vi "IMU_Single_Read_Data.vi"(8 "error in (no error)":errorcluster caption="Fehler (Eingang, kein Fehler)", 9 "Delay (ms)":u32, 11 "VISA resource name IN":refnum<visa-resource-name>) -> (0 "error out":errorcluster caption="Fehler (Ausgang)", 2 "Received Raw Data Byte-Array U8":u8[](array[numeric]), 3 "VISA resource name OUT":refnum<visa-resource-name>)   [LabVIEW 2017]
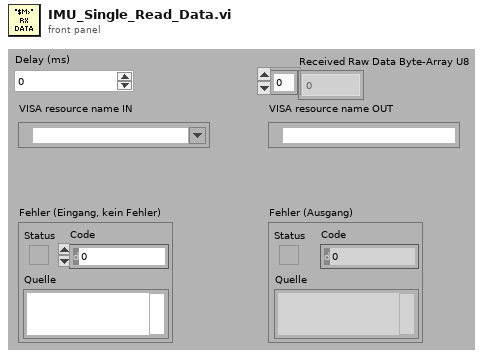
[diagram p1: front panel]
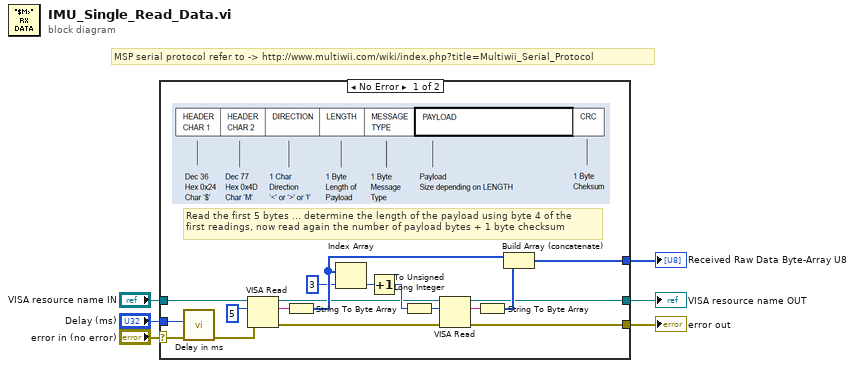
[diagram p0: block diagram]
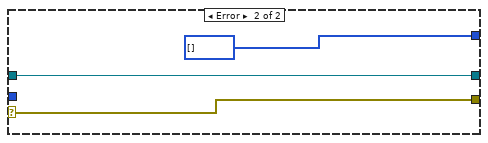
[diagram p2: hidden frame]
diagram:
  # "MSP serial protocol refer to -> http://www.multiwii.com/wiki/index.php?title=Multiwii_Serial_Protocol"
  n1 = case shown="No Error" "error in (no error)" {
    selector: "error in (no error)" -> [w24 w26]
    tunnel: "VISA resource name IN" -> [w9 w27]
    tunnel: [w11 w26] -> w5
    tunnel: [w10 w27] -> w4
    tunnel: [w8 u8[] [] ("Received Raw Data Byte-Array U8 2")] -> w3
    tunnel: "Delay (ms)" -> [w23 _]
    frame No Error {
      # "Read the first 5 bytes ... determine the length of the payload using byte 4 of the\nfirst readings, now read again the number of payload bytes + 1 byte checksum"
      n2 = call "Delay in ms.vi"("error in (no error)"=w24, "Delay Time [ms]"=w23) -> ("error out"=w7:errorcluster)  [unwired: 9 in]
      n3 = VISA Read(VISA resource name=w9, byte count=u32 5 ("Byte-Anzahl"), error in (no error)=w7) -> (VISA resource name out=w15:refnum<visa-resource-name>, read buffer=w12:string, error out=w14:errorcluster)  [unwired: 1 out]
      n4 = String To Byte Array(string=w12) -> (unsigned byte array=w21:u8[])
      n5 = Index Array(array=w21, index=3 ("Index")) -> (element=w16:u8)
      n6 = Increment(x=w16) -> (x+1=w17:u8)
      n7 = To Unsigned Long Integer(number=w17) -> (unsigned 32bit integer=w18:u32)
      n8 = VISA Read(VISA resource name=w15, byte count=w18, error in (no error)=w14) -> (VISA resource name out=w10:refnum<visa-resource-name>, read buffer=w19:string, error out=w11:errorcluster)  [unwired: 1 out]
      n9 = String To Byte Array(string=w19) -> (unsigned byte array=w20:u8[])
      n10 = Build Array (concatenate)(w21, w20) -> (w8:u8[])
    }
    frame Error {
    }
  }
  "error out" <- w5
  "VISA resource name OUT" <- w4
  "Received Raw Data Byte-Array U8" <- w3
